vi "validate fpga fxp resource type.vi"(0 "FXP Representation":T2, 11 "error in (no error)":errorcluster) -> (6 "fpga res type":T1, 8 "FXP type supported":bool, 15 "error out":errorcluster)   [LabVIEW 2017, in "FPGA Channel.lvclass"]
uses:
  FPGA Channel.lvclass
  <vilib>/fxp/LVFixedPointRepBitsTypeDef.ctl
  fpga resource supported data types.ctl
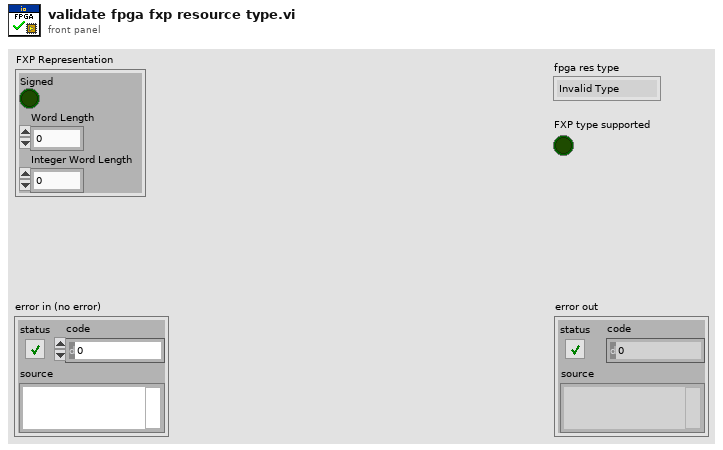
[diagram p1: front panel]
types:
  T1 = typedef "FPGA Channel.lvclass/fpga resource supported data types.ctl" = enum16{"Invalid Type", "Single", "I64", "I32", "I16", "I8", "U64", "U32", "U16", "U8", "Boolean", "FXP I,20,5", "FXP I,24,5", "FXP I,24,10", "Fifo 1023,I16"}
  T2 = typedef "LVFixedPointRepBitsTypeDef.ctl" = cluster{"Signed":bool, "Word Length":u32, "Integer Word Length":i32}
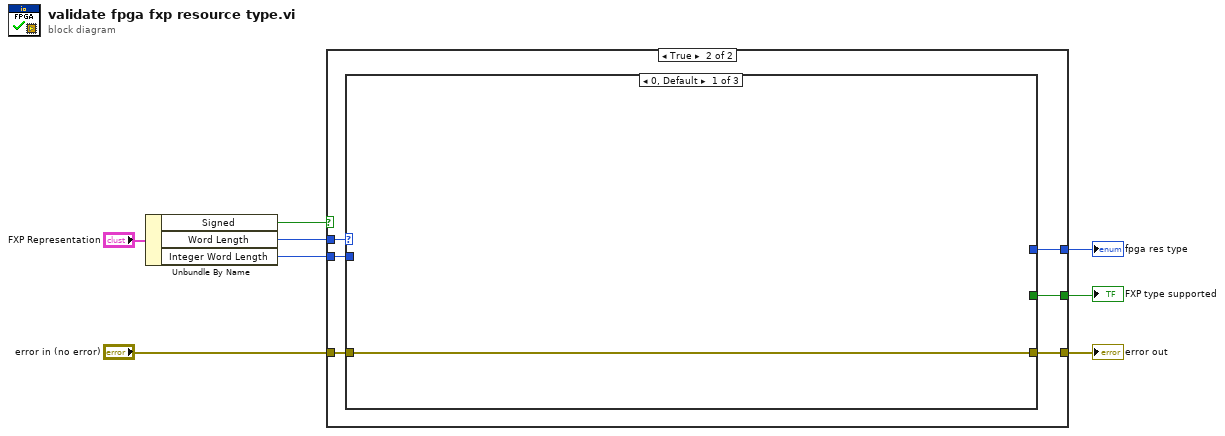
[diagram p0: block diagram]
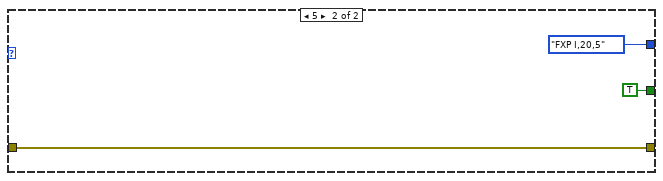
[diagram p4: hidden frame]
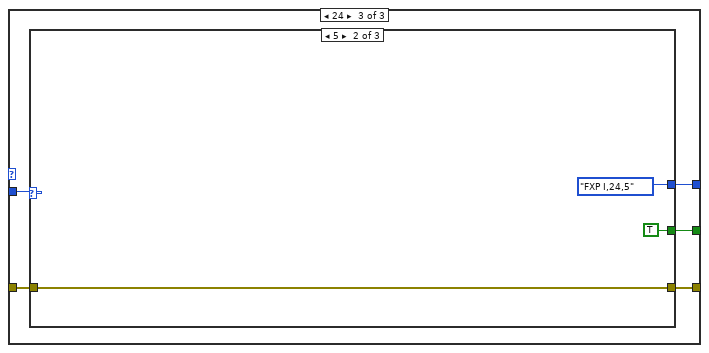
[diagram p5: hidden frame]
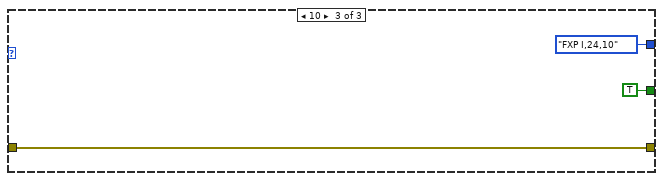
[diagram p7: hidden frame]
diagram:
  n1 = Unbundle By Name("FXP Representation") -> ("Signed"=w7:bool, "Word Length"=w6:u32, "Integer Word Length"=w5:i32)
  n2 = case shown="True" w7 {
    tunnel: w6 -> [_ w15]
    tunnel: w5 -> [_ w14]
    tunnel: "error in (no error)" -> [w9 w13]
    tunnel: [w9 w12] -> w2
    tunnel: [_ w11] -> w3
    tunnel: [_ w10] -> w1
    frame False {
    }
    frame True {
      n3 = case shown="0, Default" w15 {
        tunnel: w14 -> [_ w21 w30]
        tunnel: w13 -> [w16 w20 w29]
        tunnel: [w16 w19 w28] -> w12
        tunnel: [_ w18 w27] -> w11
        tunnel: [_ w17 w26] -> w10
        frame 0, Default {
        }
        frame 20 {
          n4 = case shown="0, Default" w21 {
            tunnel: w20 -> [w22 w24]
            tunnel: [w22 w24] -> w19
            tunnel: [_ TRUE ("FXP type supported")] -> w18
            tunnel: [_ fpga_resource_supported_data_types."FXP I,20,5" ("fpga res type")] -> w17
            frame 0, Default {
            }
            frame 5 {
            }
          }
        }
        frame 24 {
          n5 = case shown="5" w30 {
            tunnel: w29 -> [w31 w33 w36]
            tunnel: [w31 w33 w36] -> w28
            tunnel: [_ TRUE ("FXP type supported") TRUE ("FXP type supported")] -> w27
            tunnel: [_ fpga_resource_supported_data_types."FXP I,24,5" ("fpga res type") fpga_resource_supported_data_types."FXP I,24,10" ("fpga res type")] -> w26
            frame 0, Default {
            }
            frame 5 {
            }
            frame 10 {
            }
          }
        }
      }
    }
  }
  "FXP type supported" <- w3
  "error out" <- w2
  "fpga res type" <- w1
